vi "LightLoop.vi"(8 "Red Alliance":bool) -> ()   [LabVIEW 2018]
uses:
  <vilib>/Platform/TimedLoop/XDataNode/timing_clust.ctl
  <vilib>/Platform/TimedLoop/XDataNode/nitl_modes.ctl
  <vilib>/Platform/TimedLoop/XDataNode/wakeup.ctl
  <vilib>/platform/TimedLoop/XDataNode/XDataNode.xnode
  <vilib>/Platform/TimedLoop/XDataNode/XDNodeRunTimeDep.lvlib
panel:
  in  "Period (ms) 2":dbl=500.0
  in  "Duty Cycle (%) 2":dbl=50.0
  in  "Flashing":bool
  in  "Climbing":dbl=0.2
  in  "Test":bool
  in  "Period":i64=30
  in  "Duty Cycle (%)":dbl=50.0
  in  "Period (ms)":dbl=500.0
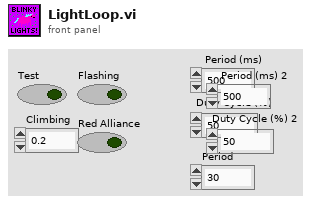
[diagram p1: front panel]
types:
  T1 = typedef "WPI_MotorControlDeviceRef.ctl" = cluster{"DeviceStatus":errorcluster, "Type":T2, "PWM":cluster{"PWM Channel":T3, "DeadBand":T4}, "CAN":cluster{"Device Number":u8, "SetOutput VI Ref":variant, "GetOutput VI Ref":variant, "Enable VI Ref":variant, "Disable VI Ref":variant, "Data":variant}, "Invert":bool, "DIO PWM":cluster{"PWM \"Enable\" Channel":T3, "DIOChannel":T5, "PWM Rate":dbl}}
  T2 = typedef "WPI_MotorControlType.ctl" = enum16{"PWM", "CAN", "DIO PWM"}
  T3 = typedef "FPGA_DIOPWMChannel.ctl" = enum8{"PWM 0", "PWM 1", "PWM 2", "PWM 3", "PWM 4", "PWM 5", "PWM 6", "PWM 7", "PWM 8", "PWM 9", "PWM MXP 0", "PWM MXP 1", "PWM MXP 2", "PWM MXP 3", "PWM MXP 4", "PWM MXP 5", "PWM MXP 6", "PWM MXP 7", "PWM MXP 8", "PWM MXP 9", "Invalid"}
  T4 = typedef "WPI_PWMDeadband.ctl" = cluster{"Name":string, "maxPositivePwm":i32, "minPositivePwm":i32, "centerPwm":i32, "maxNegativePwm":i32, "minNegativePwm":i32, "angularRange":u16}
  T5 = typedef "FPGA_DIOChannel.ctl" = enum8{"DIO 0", "DIO 1", "DIO 2", "DIO 3", "DIO 4", "DIO 5", "DIO 6", "DIO 7", "DIO 8", "DIO 9", "DIO MXP 0", "DIO MXP 1", "DIO MXP 2", "DIO MXP 3", "DIO MXP 4", "DIO MXP 5", "DIO MXP 6", "DIO MXP 7", "DIO MXP 8", "DIO MXP 9", "DIO MXP 10", "DIO MXP 11", "DIO MXP 12", "DIO MXP 13", "DIO MXP 14", "DIO MXP 15", "SPI Port CS1", "SPI Port CS2", "SPI Port CS3", "SPI Port MISO", "SPI Port MOSI", "Invalid"}
  T6 = typedef "XDNodeRunTimeDep.lvlib/timing_clust.ctl" = cluster{"Expected End [f-1]":u64, "Actual End [f-1]":u64, "Finished Late? [f-1]":bool, "Expected End [i-1]":u64, "Actual End [i-1]":u64, "Finished Late? [i-1]":bool, "Expected Start [i]":u64, "Actual Start [i]":u64, "Expected Start [f]":u64, "Actual Start [f]":u64, "Source Name":string, "Structure Name":string, "Period":i64, "Deadline":i64, "Offset":i64, "Start":i64, "Priority":i32, "Timeout":i32, "Mode":T7, "Wakeup Reason":T8, "Error":errorcluster, "Source Type":string, "Secondary Source Type":string, "Global End Time":u64, "Global Start Time":u64, "Frame Duration":u64, "Iteration Duration":u64, "Assigned CPU":i32, "I/O Scan Engine Mode":u32}
  T7 = typedef "XDNodeRunTimeDep.lvlib/nitl_modes.ctl" = enum32{"No Change", "Process missed periods, maintain original phase", "Discard missed periods, maintain original phase", "Process missed periods, ignore original phase", "Discard missed periods, ignore original phase"}
  T8 = typedef "XDNodeRunTimeDep.lvlib/wakeup.ctl" = enum32{"Normal", "Aborted", "Asynchronous wakeup", "Timing source error", "Timed loop error", "Timeout"}
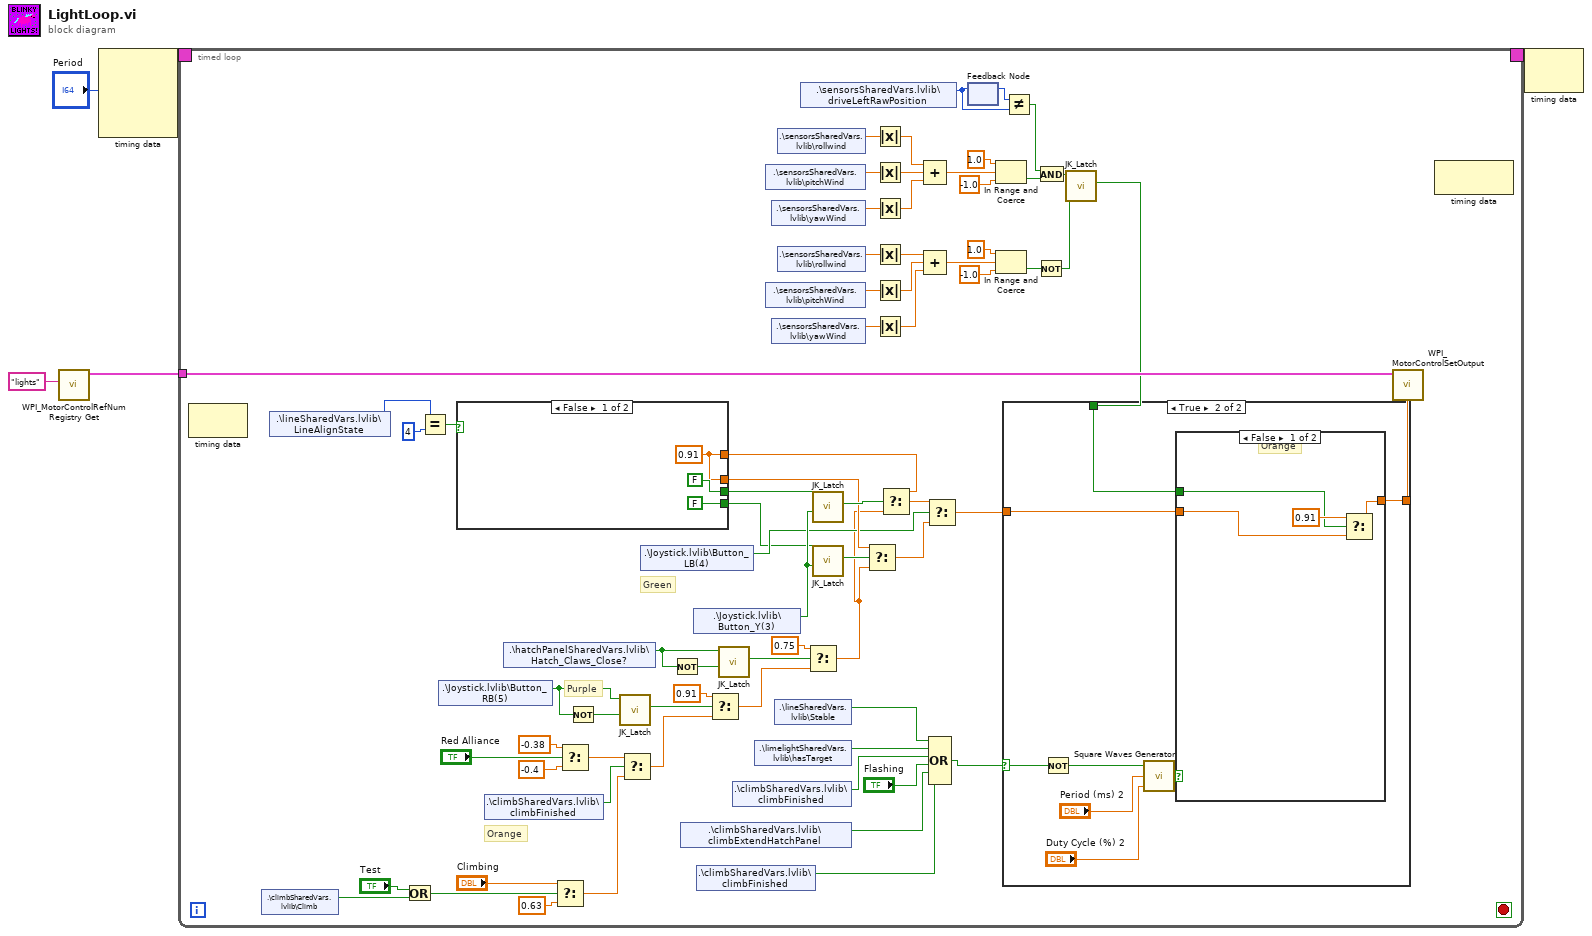
[diagram p0: block diagram]
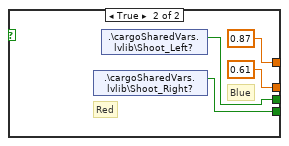
[diagram p2: hidden frame]
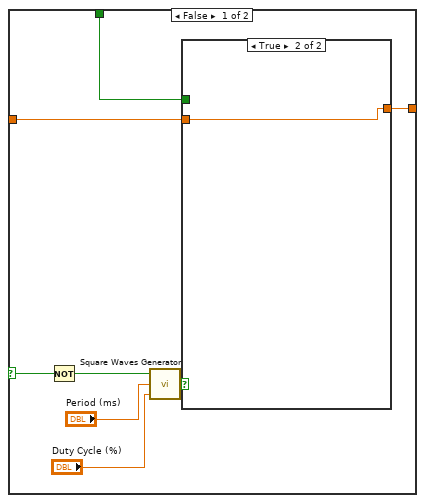
[diagram p3: hidden frame]
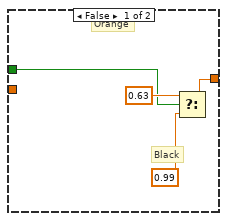
[diagram p4: hidden frame]
diagram:
  n1 = call <vilib>:"WPI_MotorControlRefNum Registry Get.vi"("refnum name"="lights") -> ("MotorControlDevRef"=w2:T1)  [unwired: 9 in, 1 out]
  n2 = node-c288("Period") -> (w5:T6)  [unwired: 3 in]
  n3 = timed-loop {
    timing: w5 -> [_]
    timing-out: [_] -> w4
    tunnel: w2 -> [w68]
    stop <- _ stop-if-true
    # "Orange"
    # "Purple"
    # "Green"
    n4 = node-c288() -> ()  [unwired: 1 in, 1 out]
    n5 = shared-variable ".\\climbSharedVars.lvlib\\Climb"() -> (w58:bool)  [unwired: 1 in, 1 out]
    n6 = shared-variable ".\\lineSharedVars.lvlib\\LineAlignState"() -> (w42:i32)  [unwired: 1 in, 1 out]
    n7 = Or(x="Test", y=w58) -> (x .or. y?=w57:bool)
    n8 = Equal?(x=w42, y=4) -> (x = y?=w43:bool)
    n9 = shared-variable ".\\Joystick.lvlib\\Button_RB(5)"() -> (w46:bool)  [unwired: 1 in, 1 out]
    n10 = case shown="False" w43 {
      tunnel: [FALSE ("Boolean") w83] -> w33
      tunnel: [FALSE ("Boolean") w82] -> w34
      tunnel: [w77 0.61 ("t")] -> w40
      tunnel: [w77 0.87 ("t")] -> w39
      frame False {
        w77 = 0.91 ("t")
      }
      frame True {
        # "Blue"
        # "Red"
        n11 = shared-variable ".\\cargoSharedVars.lvlib\\Shoot_Right?"() -> (w83:bool)  [unwired: 1 in, 1 out]
        n12 = shared-variable ".\\cargoSharedVars.lvlib\\Shoot_Left?"() -> (w82:bool)  [unwired: 1 in, 1 out]
      }
    }
    n13 = shared-variable ".\\climbSharedVars.lvlib\\climbFinished"() -> (w61:bool)  [unwired: 1 in, 1 out]
    n14 = shared-variable ".\\hatchPanelSharedVars.lvlib\\Hatch_Claws_Close?"() -> (w44:bool)  [unwired: 1 in, 1 out]
    n15 = Select(t="Climbing", s=w57, f=0.63) -> (s? t:f=w59:dbl)
    n16 = Select(t=-0.38, s="Red Alliance", f=-0.4) -> (s? t:f=w51:dbl)
    n17 = Not(x=w46) -> (.not. x?=w47:bool)
    n18 = call <userlib>:"JK_Latch.vi"("Reset"=w47, "Set"=w46) -> ("Q"=w64:bool)  [unwired: 5 in]
    n19 = Select(t=w51, s=w61, f=w59) -> (s? t:f=w62:dbl)
    n20 = shared-variable ".\\Joystick.lvlib\\Button_LB(4)"() -> (w35:bool)  [unwired: 1 in, 1 out]
    n21 = Not(x=w44) -> (.not. x?=w45:bool)
    n22 = shared-variable ".\\climbSharedVars.lvlib\\climbExtendHatchPanel"() -> (w52:bool)  [unwired: 1 in, 1 out]
    n23 = shared-variable ".\\Joystick.lvlib\\Button_Y(3)"() -> (w65:bool)  [unwired: 1 in, 1 out]
    n24 = shared-variable ".\\climbSharedVars.lvlib\\climbFinished"() -> (w38:bool)  [unwired: 1 in, 1 out]
    n25 = Select(t=0.91, s=w64, f=w62) -> (s? t:f=w75:dbl)
    n26 = call <userlib>:"JK_Latch.vi"("Reset"=w45, "Set"=w44) -> ("Q"=w63:bool)  [unwired: 5 in]
    n27 = shared-variable ".\\climbSharedVars.lvlib\\climbFinished"() -> (w54:bool)  [unwired: 1 in, 1 out]
    n28 = shared-variable ".\\limelightSharedVars.lvlib\\hasTarget"() -> (w70:bool)  [unwired: 1 in, 1 out]
    n29 = shared-variable ".\\sensorsSharedVars.lvlib\\pitchWind"() -> (w24:dbl)  [unwired: 1 in, 1 out]
    n30 = shared-variable ".\\sensorsSharedVars.lvlib\\pitchWind"() -> (w20:dbl)  [unwired: 1 in, 1 out]
    n31 = shared-variable ".\\sensorsSharedVars.lvlib\\yawWind"() -> (w23:dbl)  [unwired: 1 in, 1 out]
    n32 = shared-variable ".\\sensorsSharedVars.lvlib\\yawWind"() -> (w19:dbl)  [unwired: 1 in, 1 out]
    n33 = shared-variable ".\\lineSharedVars.lvlib\\Stable"() -> (w71:bool)  [unwired: 1 in, 1 out]
    n34 = shared-variable ".\\sensorsSharedVars.lvlib\\rollwind"() -> (w29:dbl)  [unwired: 1 in, 1 out]
    n35 = shared-variable ".\\sensorsSharedVars.lvlib\\rollwind"() -> (w22:dbl)  [unwired: 1 in, 1 out]
    n36 = shared-variable ".\\sensorsSharedVars.lvlib\\driveLeftRawPosition"() -> (w26:i32)  [unwired: 1 in, 1 out]
    n37 = Select(t=0.75, s=w63, f=w75) -> (s? t:f=w32:dbl)
    n38 = call <userlib>:"JK_Latch.vi"("Reset"=w65, "Set"=w34) -> ("Q"=w66:bool)  [unwired: 5 in]
    n39 = call <userlib>:"JK_Latch.vi"("Reset"=w65, "Set"=w33) -> ("Q"=w67:bool)  [unwired: 5 in]
    n40 = Select(t=w40, s=w67, f=w32) -> (s? t:f=w36:dbl)
    n41 = Absolute Value(x=w29) -> (abs(x)=w6:dbl)
    n42 = Absolute Value(x=w24) -> (abs(x)=w7:dbl)
    n43 = Absolute Value(x=w23) -> (abs(x)=w8:dbl)
    n44 = Absolute Value(x=w22) -> (abs(x)=w9:dbl)
    n45 = Absolute Value(x=w20) -> (abs(x)=w10:dbl)
    n46 = Absolute Value(x=w19) -> (abs(x)=w11:dbl)
    n47 = Select(t=w39, s=w66, f=w32) -> (s? t:f=w76:dbl)
    n48 = Compound Arithmetic op=ADD(w6, w7, w8) -> (w25:dbl)
    n49 = Compound Arithmetic op=ADD(w9, w10, w11) -> (w21:dbl)
    n50 = Select(t=w76, s=w35, f=w36) -> (s? t:f=w37:dbl)
    n51 = Compound Arithmetic op=OR(w71, w70, w54, "Flashing", w52, w38) -> (w72:bool)
    n52 = feedback-in #1(w26) -> ()
    n53 = feedback #1() -> (w27:i32)  [unwired: 1 in]
    n54 = In Range and Coerce(upper limit=1.0, x=w25, lower limit=-1.0) -> (In Range?=w30:bool)  [unwired: 1 out]
    n55 = In Range and Coerce(upper limit=1.0, x=w21, lower limit=-1.0) -> (In Range?=w18:bool)  [unwired: 1 out]
    n56 = Not Equal?(x=w27, y=w26) -> (x != y?=w28:bool)
    n57 = Not(x=w18) -> (.not. x?=w15:bool)
    n58 = And(x=w28, y=w30) -> (x .and. y?=w31:bool)
    n59 = call <userlib>:"JK_Latch.vi"("Reset"=w15, "Set"=w31) -> ("Q"=w17:bool)  [unwired: 5 in]
    n60 = case shown="True" w72 {
      selector: w72 -> [w90 w103]
      tunnel: w37 -> [w88 w101]
      tunnel: [w87 w100] -> w69
      tunnel: w17 -> [w84 w97]
      frame False {
        n61 = Not(x=w90) -> (.not. x?=w89:bool)
        n62 = call <userlib>:"Square Waves Generator.vi"("Duty Cycle (%)"="Duty Cycle (%)", "Period (ms)"="Period (ms)", "Enable"=w89) -> ("Signal"=w91:bool)
        n63 = case shown="True" w91 {
          tunnel: w88 -> [_ w96]
          tunnel: [w94 w96] -> w87
          tunnel: w84 -> [w92 _]
          frame False {
            # "Orange"
            # "Black"
            n64 = Select(t=0.63 ("f"), s=w92, f=0.99) -> (s? t:f=w94:dbl)
          }
          frame True {
          }
        }
      }
      frame True {
        n65 = Not(x=w103) -> (.not. x?=w102:bool)
        n66 = call <userlib>:"Square Waves Generator.vi"("Duty Cycle (%)"="Duty Cycle (%) 2", "Period (ms)"="Period (ms) 2", "Enable"=w102) -> ("Signal"=w104:bool)
        n67 = case shown="False" w104 {
          tunnel: w101 -> [w105 w109]
          tunnel: [w108 w109] -> w100
          tunnel: w97 -> [w106 _]
          frame False {
            # "Orange"
            n68 = Select(t=0.91 ("f"), s=w106, f=w105) -> (s? t:f=w108:dbl)
          }
          frame True {
          }
        }
      }
    }
    n69 = call <vilib>:"WPI_MotorControlSetOutput.vi"("Output"=w69, "MotorControlDevRef"=w68) -> ()  [unwired: 7 in, 3 out]
    n70 = node-c288() -> ()  [unwired: 1 in, 1 out]
  }
  n71 = node-c288(w4) -> ()  [unwired: 1 out]
